vi "Actor Core.vi"(8 "error in":errorcluster, 11 "PID Controller in":refnum<class "PID Controller.lvclass">) -> (0 "error out":errorcluster, 3 "Actor out":refnum<class "Actor.lvclass">)   [LabVIEW 2024, in "PID Controller.lvlib" / "PID Controller.lvclass"]
doc: "<p>(<strong>Filename</strong>: <span class=\"dnl\">Actor Framework.lvlib:Actor.lvclass:Actor Core.vi</span>)</p>\n<p>Receives messages to the actor, reacts to them, and initiates any error handling that may shut the actor down.</p>\n<p>Descendant classes may override this VI to append parallel tasks for the actor to complete while it handles messages. Overrides use the <a href=\"nihelplauncher://docs/csh?context=lvcore_glang_udclass\">Call Parent Class Method</a> node.</p>"
uses:
  PID Controller.lvclass
  <vilib>/ActorFramework/Actor/Actor.lvclass
  PID Controller.lvclass/PID Controller.ctl
panel:
  out "Waveform Chart":dbl(graph)
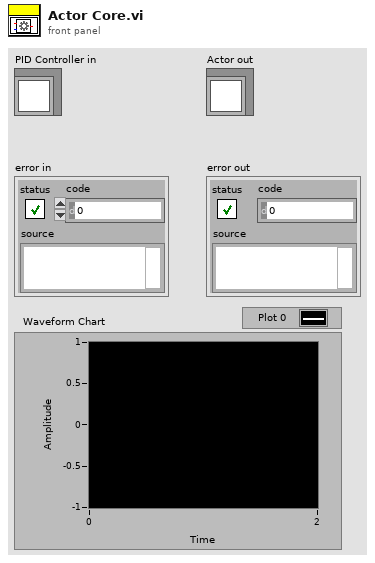
[diagram p1: front panel]
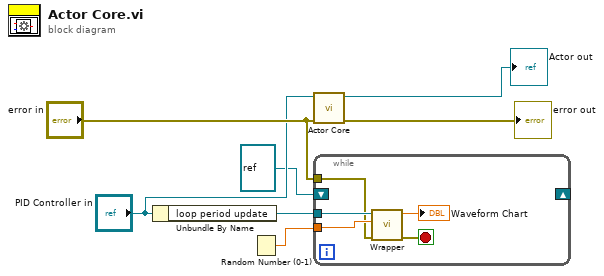
[diagram p0: block diagram]
diagram:
  n1 = Unbundle By Name("PID Controller in") -> ("loop period update"=w3:refnum<notifier>)
  n2 = Random Number (0-1)() -> (number: 0 to 1=w2:dbl)
  n3 = call-parent "Actor Core.vi"("error in"="error in", "Actor in"="PID Controller in") -> ("error out"=→"error out":errorcluster, "Actor out"=→"Actor out":refnum<class "Actor.lvclass">)  [unwired: 8 in]
  n4 = while {
    tunnel: "error in" -> [w10]
    tunnel: w3 -> [w12]
    tunnel: w2 -> [w11]
    shift-right: _ -> [_]
    shift-left: refnum<vi> refnum ("vi reference") -> [_]
    stop <- w9 stop-if-true
    n5 = call "Wrapper.vi"("error in (no error)"=w10, "setpoint"=w11, "loop period update"=w12) -> ("error out"=w9:errorcluster, "output"=→"Waveform Chart":dbl)  [unwired: 7 in]
  }
